vi "Downhill Simplex nD.vi"(4 "f(X)":string, 5 "X":string[](array[string]), 6 "Start":dbl[](array[numeric]) format="%.2f", 7 "accuracy":dbl=1e-08 format="%.2e") -> (0 "error":i32, 1 "ticks":u32, 2 "f(Minimum)":dbl format="%.2f", 3 "Minimum":dbl[](array[numeric]) format="%.2f")   [LabVIEW 2018, in "NI_Gmath.lvlib"]
doc: "Determines a local minimum of a function of n independent variables with the Downhill Simplex method."
uses:
  NI_Gmath.lvlib
panel:
  # "Example:\n\n accuracy: 1E-8 \n Start: 0.0 and 0.0 \n X: x and y\n f(X): x^2+y^2+sin(x-y)"
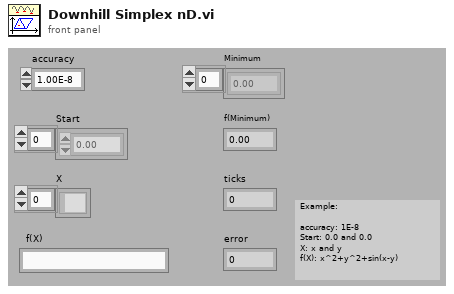
[diagram p1: front panel]
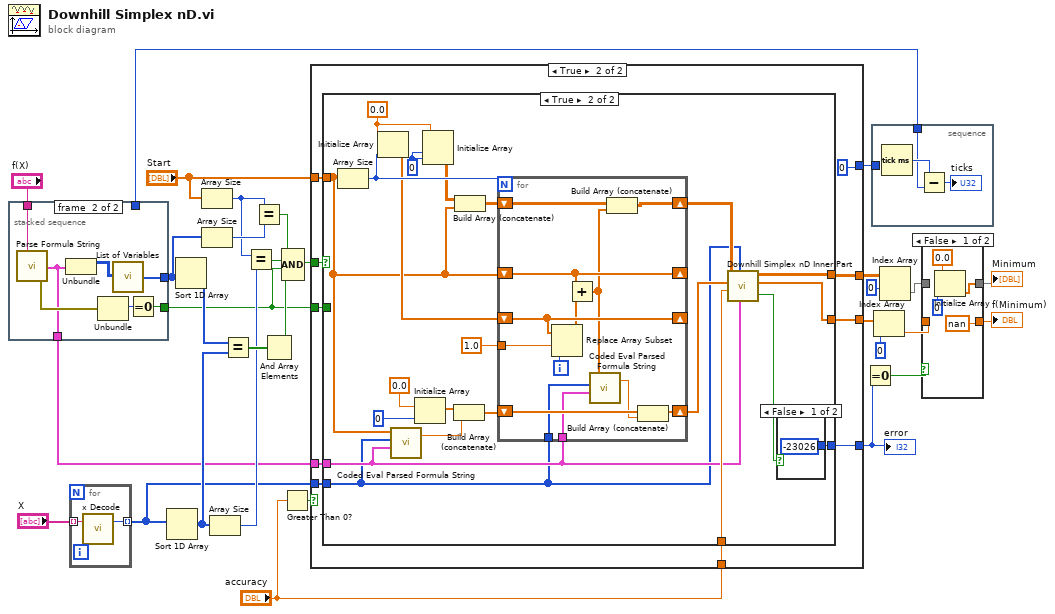
[diagram p0: block diagram]
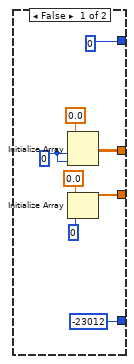
[diagram p3: hidden frame]
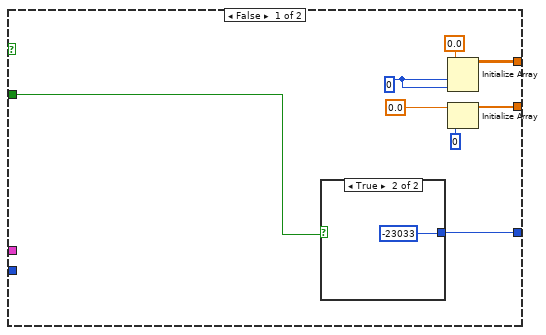
[diagram p4: hidden frame]
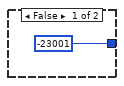
[diagram p5: hidden frame]
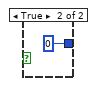
[diagram p6: hidden frame]
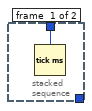
[diagram p7: hidden frame]
diagram:
  n1 = stacked-sequence {
    tunnel: [_ w39] -> w6
    tunnel: [w32 _] -> w30
    tunnel: [_ w38] -> w27
    tunnel: "f(X)" -> [_ w37]
    tunnel: [_ w33] -> w2
    frame #0 {
      n2 = Tick Count (ms)() -> (millisecond timer value=w32:u32)
    }
    frame #1 {
      n3 = call "Parse Formula String.vi"("formula"=w37) -> ("error out"=w36:errorcluster, "Parsed Formula"=w33:cluster{"Table":i32[][], "Y Values":dbl[]})  [unwired: 1 in]
      n4 = Unbundle(w33) -> ("Table"=w35:i32[][])  [unwired: 1 out]
      n5 = Unbundle(w36) -> ("code"=w34:i32)  [unwired: 2 out]
      n6 = call "List of Variables.vi"("Table"=w35) -> ("List of variables"=w38:i32[])
      n7 = Equal To 0?(x=w34) -> (x = 0?=w39:bool)
    }
  }
  n8 = for {
    tunnel: "X" -> [w41] mode=indexing
    tunnel: [w40] -> w1 mode=indexing
    n9 = call "x Decode.vi"("x string"=w41) -> ("number"=w40:i32)  [unwired: 1 in, 1 out]
  }
  n10 = Sort 1D Array(array=w1) -> (sorted array=w9:i32[])
  n11 = Sort 1D Array(array=w27) -> (sorted array=w25:i32[])
  n12 = Array Size(array="Start") -> (size(s)=w8:i32)
  n13 = Array Size(array=w27) -> (size(s)=w26:i32)
  n14 = Array Size(array=w9) -> (size(s)=w7:i32)
  n15 = Equal?(x=w25, y=w9) -> (x = y?=w24:bool[])
  n16 = Equal?(x=w8, y=w7) -> (x = y?=w4:bool)
  n17 = Equal?(x=w8, y=w26) -> (x = y?=w5:bool)
  n18 = And Array Elements(Boolean array=w24) -> (logical AND=w23:bool)
  n19 = Compound Arithmetic op=AND(w5, w4, w6, w23) -> (w3:bool)
  n20 = Greater Than 0?(x="accuracy") -> (x > 0?=w17:bool)
  n21 = case shown="True" w17 {
    tunnel: [w43 w59] -> w19
    tunnel: [w44 w58] -> w20
    tunnel: "accuracy" -> [_ w57]
    tunnel: "Start" -> [_ w56]
    tunnel: [0 0] -> w31
    tunnel: [-23012 w54] -> w16
    tunnel: w6 -> [_ w53]
    tunnel: w3 -> [_ w52]
    tunnel: w2 -> [_ w51]
    tunnel: w1 -> [_ w50]
    frame False {
      w47 = 0
      n22 = Initialize Array(0.0, w47, w47) -> (w44:dbl[][])
      n23 = Initialize Array(0.0, 0) -> (w43:dbl[])
    }
    frame True {
      n24 = case shown="True" w52 {
        tunnel: w56 -> [_ w77]
        tunnel: w57 -> [_ w74]
        tunnel: [w63 w73] -> w58
        tunnel: [w62 w72] -> w59
        tunnel: [w61 w80] -> w54
        tunnel: w53 -> [w60 _]
        tunnel: w51 -> [_ w71]
        tunnel: w50 -> [_ w70]
        frame False {
          w66 = 0
          n25 = case shown="True" w60 {
            tunnel: [-23001 -23033] -> w61
            frame False {
            }
            frame True {
            }
          }
          n26 = Initialize Array(0.0, w66, w66) -> (w63:dbl[][])
          n27 = Initialize Array(0.0, 0) -> (w62:dbl[])
        }
        frame True {
          w83 = 0.0
          w87 = 0
          n28 = Array Size(array=w77) -> (size(s)=w86:i32)
          n29 = Initialize Array(w83, w86) -> (w82:dbl[])
          n30 = call "Coded Eval Parsed Formula String.vi"("Parsed Formula"=w71, "Variables"=w70, "X Values"=w77) -> ("y value"=w76:dbl)  [unwired: 1 in, 1 out]
          n31 = Initialize Array(0.0, 0) -> (w90:dbl[])
          n32 = Initialize Array(w83, w87, w87) -> (w84:dbl[][])
          n33 = Build Array (concatenate)(w90, w76) -> (w91:dbl[])
          n34 = Build Array (concatenate)(w84, w77) -> (w85:dbl[][])
          n35 = for {
            N: w86 -> [_]
            shift-right: [w105] -> w79
            shift-left: w85 -> [w106]
            shift-right: [w101] -> _
            shift-left: w77 -> [w101]
            shift-right: [w104] -> _
            shift-left: w82 -> [w104]
            tunnel: 1.0 -> [w98]
            shift-right: [w102] -> w75
            shift-left: w91 -> [w103]
            tunnel: w71 -> [w95]
            tunnel: w70 -> [w96]
            i -> [w99]
            n36 = Replace Array Subset(array=w104, new element=w98, index=w99) -> (w100:dbl[])
            n37 = Add(x=w101, y=w100) -> (x+y=w97:dbl[])
            n38 = call "Coded Eval Parsed Formula String.vi"("Parsed Formula"=w95, "Variables"=w96, "X Values"=w97) -> ("y value"=w94:dbl)  [unwired: 1 in, 1 out]
            n39 = Build Array (concatenate)(w106, w97) -> (w105:dbl[][])
            n40 = Build Array (concatenate)(w103, w94) -> (w102:dbl[])
          }
          n41 = call "Downhill Simplex nD Inner Part.vi"("Parsed Formula"=w71, "Variables"=w70, "accuracy"=w74, "f(Minimum) before"=w75, "Minimum before"=w79) -> ("f(Minimum) after"=w72:dbl[], "Minimum after"=w73:dbl[][], "convergence"=w81:bool)  [unwired: 4 in]
          n42 = case shown="False" w81 {
            tunnel: [-23026 0] -> w80
            frame False {
            }
            frame True {
            }
          }
        }
      }
    }
  }
  "error" <- w16
  n43 = Equal To 0?(x=w16) -> (x = 0?=w15:bool)
  n44 = stacked-sequence {
    tunnel: w30 -> [w108]
    tunnel: w31 -> [_]
    frame #0 {
      n45 = Tick Count (ms)() -> (millisecond timer value=w109:u32)
      n46 = Subtract(x=w109, y=w108) -> (x-y=→"ticks":u32)
    }
  }
  n47 = Index Array(array=w19, index=0) -> (element=w12:dbl)
  n48 = Index Array(array=w20, index (row)=0) -> (element=w14:dbl[])  [unwired: 1 in]
  n49 = case shown="False" w15 {
    tunnel: w14 -> [_ w115]
    tunnel: [w110 w115] -> w13
    tunnel: w12 -> [_ w114]
    tunnel: [nan w114] -> w11
    frame False {
      n50 = Initialize Array(0.0, 0) -> (w110:dbl[])
    }
    frame True {
    }
  }
  "Minimum" <- w13
  "f(Minimum)" <- w11
